vi "exp seq init logic.vi"(0 "proceed":bool, 1 "exp exec in":T1={"data file"={"autosave"=FALSE, "File refnum"=refnum, "data file path"=path ""}, "T log file"={"File refnum"=refnum, "T log file path"=path "", "exists"=FALSE}, "exp seq"={"wave params"={"Num of avg"=0, "Num points"=1000, "Meas rate (Hz)"=100000.0}, "Setpoints"=[], "#"=-1, "index"=-1, "elapsed time (s)"=0.0, "set time (s)"=0.0, "min settle (s)"=30.0, " Exec Status"=enum."Settling"}, "error"={"status"=FALSE, "code"=0, "source"=""}}, 7 "x":bool, 11 "exit":bool) -> (4 "stop loop":bool, 15 "Experimental Sequence":T7)   [LabVIEW 2019]
doc: "This subVI is just a convienience. It encapsulates some space filling exit logic for the initialization phase of the executive loop.\n\nPaul K Dixon\nP3600\nCSUSB Physics"
uses:
  typedefs/exp sequence.ctl
  typedefs/PID exec cluster.ctl
  typedefs/data file info.ctl
  typedefs/bug temp file info.ctl
  typedefs/exp seq cluster.ctl
  typedefs/wvfm acq params.ctl
  typedefs/bug meas status.ctl
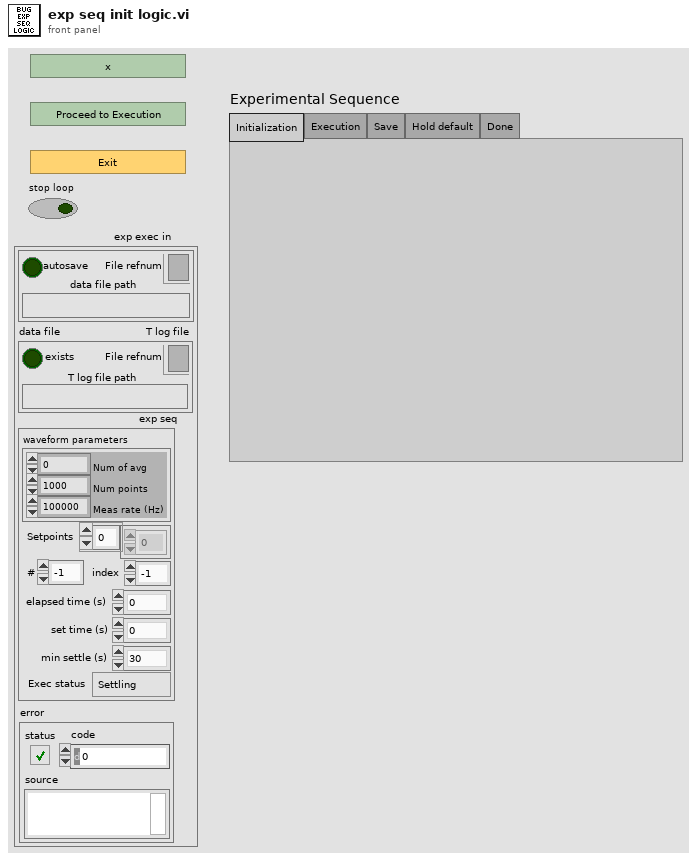
[diagram p1: front panel]
types:
  T1 = typedef "PID exec cluster.ctl" = cluster{"data file":T2, "T log file":T3, "exp seq":T4, "error":errorcluster}
  T2 = typedef "data file info.ctl" = cluster{"autosave":bool, "File refnum":refnum<file>, "data file path":path}
  T3 = typedef "bug temp file info.ctl" = cluster{"File refnum":refnum<file>, "T log file path":path, "exists":bool}
  T4 = typedef "exp seq cluster.ctl" = cluster{"wave params":T5, "Setpoints":dbl[], "#":i32, "index":i32, "elapsed time (s)":dbl, "set time (s)":dbl, "min settle (s)":dbl, " Exec Status":T6}
  T5 = typedef "wvfm acq params.ctl" = cluster{"Num of avg":i32, "Num points":i32, "Meas rate (Hz)":dbl}
  T6 = typedef "bug meas status.ctl" = enum32{"Settling", "Measuring", "Holding", "Exit"}
  T7 = typedef "exp sequence.ctl" = enum32{"Initialization", "Execution", "Save", "Hold default", "Done"}
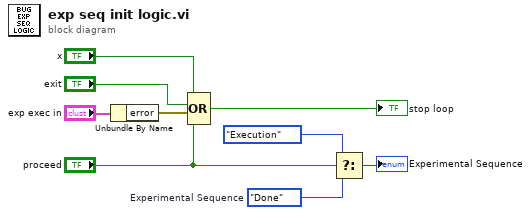
[diagram p0: block diagram]
diagram:
  w6 = exp_sequence."Done"  # Experimental Sequence
  n1 = Unbundle By Name("exp exec in") -> ("error"=w3:errorcluster)
  n2 = Compound Arithmetic op=OR("x", "exit", w3, "proceed") -> (→"stop loop":bool)
  n3 = Select(t=exp_sequence."Execution" ("Experimental Sequence"), s="proceed", f=w6) -> (s? t:f=→"Experimental Sequence":T7)
